vi "Read Write datanew.vi"(7 "Enum":T2(ring), 8 "error in":errorcluster, 10 "Data In":T1(array[cluster]), 11 "appended path":path) -> (0 "error out":errorcluster, 2 "data out":T1(array[cluster]))   [LabVIEW 2013]
doc: "This subVI reads the data from ATM account.txt"
uses:
  <vilib>/Utility/file.llb/Read From Spreadsheet File (string).vi
  <vilib>/Utility/file.llb/Write To Spreadsheet File (string).vi
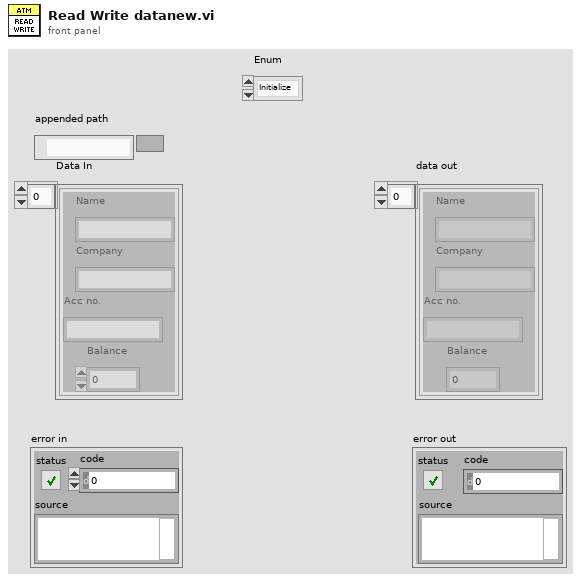
[diagram p1: front panel]
types:
  T1 = cluster{"Name":string, "Company":string, "Acc no.":string, "Balance":i32}[]
  T2 = enum16{"Initialize", "Read", "Write", "Process", "Stop"}
  T3 = cluster{"Name":string, "Company":string, "Acc no.":string, "Balance":i32}
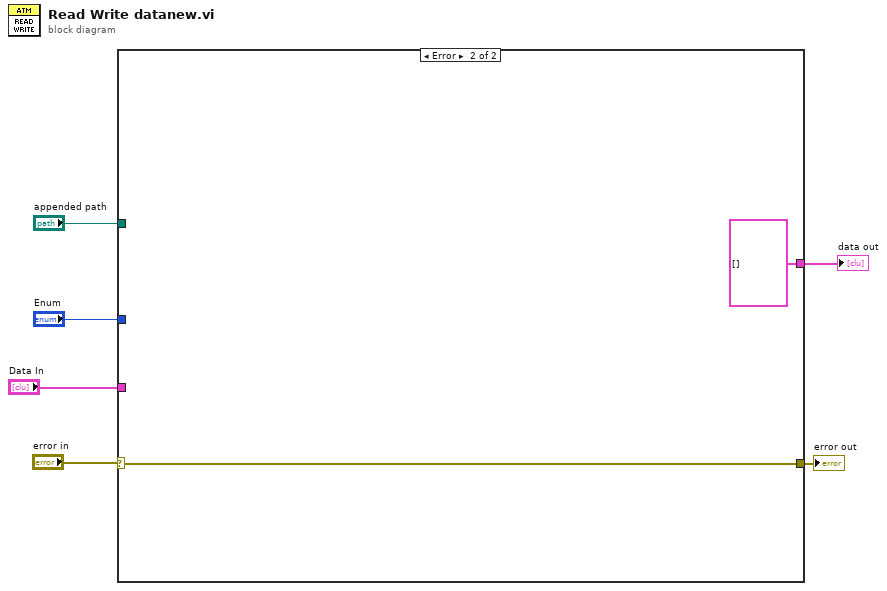
[diagram p0: block diagram]
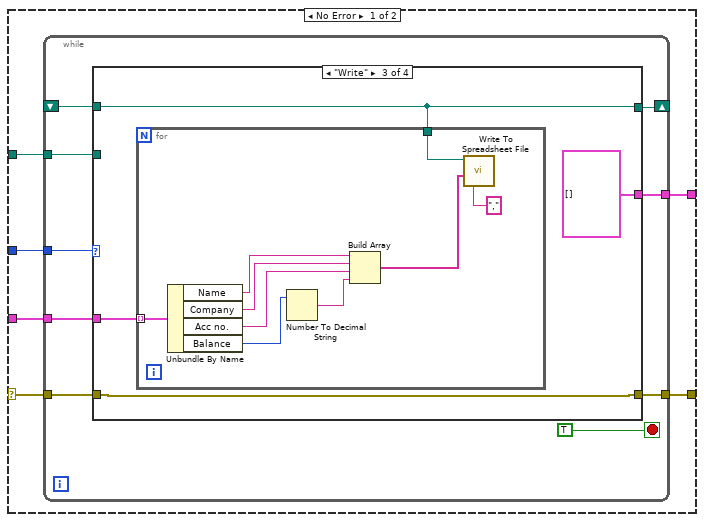
[diagram p2: hidden frame]
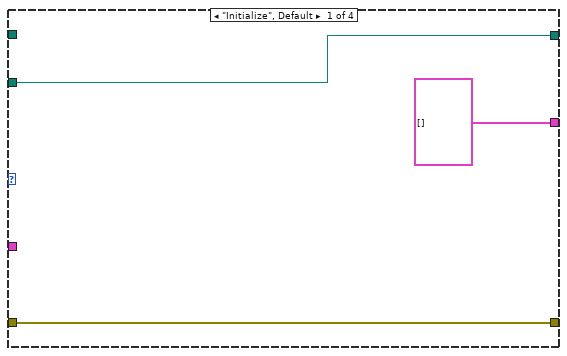
[diagram p3: hidden frame]
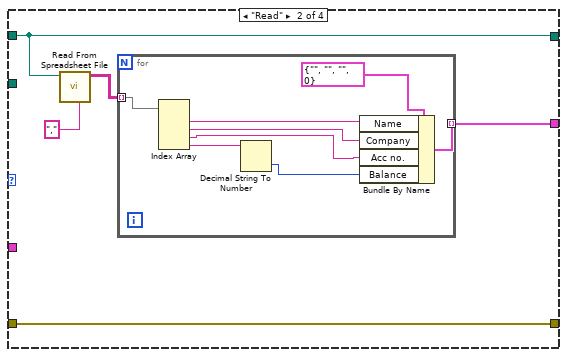
[diagram p4: hidden frame]
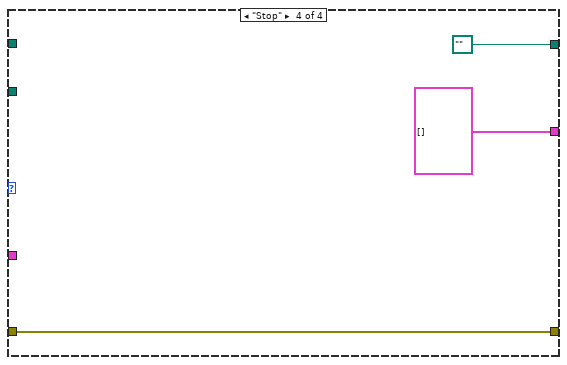
[diagram p5: hidden frame]
diagram:
  n1 = case shown="Error" "error in" {
    selector: "error in" -> [w10 w55]
    tunnel: "appended path" -> [w12 _]
    tunnel: "Enum" -> [w11 _]
    tunnel: [w9 w55] -> w3
    tunnel: [w8 T1 []] -> w2
    tunnel: "Data In" -> [w7 _]
    frame No Error {
      n2 = while {
        tunnel: w11 -> [w21]
        tunnel: w12 -> [w20]
        shift-right: [w19] -> _
        shift-left: _ -> [w18]
        tunnel: w10 -> [w17]
        tunnel: [w16] -> w9
        tunnel: [w14] -> w8
        tunnel: w7 -> [w13]
        stop <- TRUE stop-if-true
        n3 = case shown="\"Write\"" w21 {
          tunnel: w20 -> [w24 _ _ _]
          tunnel: [w24 w29 w39 path "" ("appended path")] -> w19
          tunnel: w18 -> [_ w29 w39 _]
          tunnel: w17 -> [w23 w27 w38 w52]
          tunnel: [w23 w27 w38 w52] -> w16
          tunnel: [T1 [] w25 T1 [] T1 []] -> w14
          tunnel: w13 -> [_ _ w41 _]
          frame "Initialize", Default {
          }
          frame "Read" {
            n4 = call-poly <vilib>:"Read From Spreadsheet File.vi"("delimiter (\\t)"="," ("delimiter (\\t)"), "file path (dialog if empty)"=w29) -> ("all rows"=w28:string[][])  [unwired: 5 in, 4 out]
            n5 = for {
              tunnel: w28 -> [w37] mode=indexing
              tunnel: [w35] -> w25 mode=indexing
              n6 = Index Array(array=w37) -> (element #1=w33:string, element #2=w32:string, element #3=w31:string, element #4=w36:string)  [unwired: 4 in]
              n7 = Decimal String To Number(string=w36) -> (number=w30:i32)  [unwired: 2 in, 1 out]
              n8 = Bundle By Name(cluster=T3 {"Name"="", "Company"="", "Acc no."="", "Balance"=0} ("data out"), "Name"=w33, "Company"=w32, "Acc no."=w31, "Balance"=w30) -> (w35:T3)
            }
          }
          frame "Write" {
            n9 = for {
              tunnel: w41 -> [w50] mode=indexing
              tunnel: w39 -> [w42]
              n10 = Unbundle By Name(w50) -> ("Name"=w49:string, "Company"=w48:string, "Acc no."=w47:string, "Balance"=w46:i32)
              n11 = Number To Decimal String(number=w46) -> (decimal integer string=w45:string)  [unwired: 1 in]
              n12 = Build Array(w49, w48, w47, w45) -> (w44:string[])
              n13 = call-poly <vilib>:"Write To Spreadsheet File.vi"("delimiter (\\t)"="," ("delimiter (\\t)"), "1D data"=w44, "file path (dialog if empty)"=w42) -> ()  [unwired: 5 in, 1 out]
            }
          }
          frame "Stop" {
          }
        }
      }
    }
    frame Error {
    }
  }
  "error out" <- w3
  "data out" <- w2
